vi "Mean Demo.vi"() -> ()   [LabVIEW 2012]
panel:
  out "平均值":dbl
  out "随机数图表":cluster{"number: 0 to 1":dbl, "mean":dbl}(graph)
  in  "停止":bool
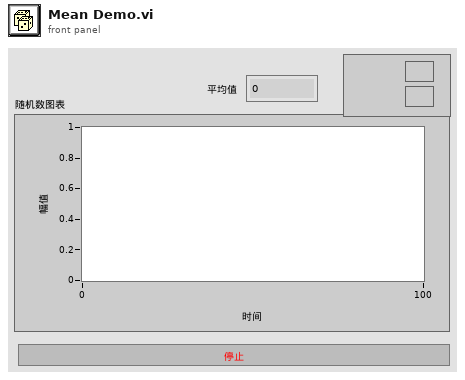
[diagram p1: front panel]
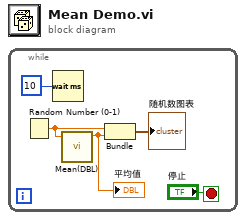
[diagram p0: block diagram]
diagram:
  n1 = while {
    stop <- "停止" stop-if-true
    n2 = Random Number (0-1)() -> (number: 0 to 1=w4:dbl)
    n3 = Wait (ms)(milliseconds to wait=u32 10 ("等待时间（毫秒）")) -> ()  [unwired: 1 out]
    n4 = call "Mean(DBL).vi"("input"=w4) -> ("mean"=w3:dbl)  [unwired: 9 in, 1 out]
    "平均值" <- w3
    n5 = Bundle("number: 0 to 1"=w4, "mean"=w3) -> (→"随机数图表":cluster{"number: 0 to 1":dbl, "mean":dbl})  [unwired: 1 in]
  }
